vi "Preset GB VOLTAGE.vi"(8 "error in (no error)":errorcluster, 10 "Voltage":dbl=1.0 min=1.0 max=8.0 step=0.1 format="%.1f", 11 "VISA resource in":refnum<visa-resource-name>) -> (0 "error out":errorcluster, 3 "VISA resource out":refnum<visa-resource-name>)   [LabVIEW 2025, in "Chroma 19572.lvlib"]
doc: "This VI writes to the instrument the GFI state."
uses:
  <instrlib>/Chroma 19572/Chroma 19572.lvlib
panel:
  # "PreSet GB VOLTAGE"
  # "[V]"
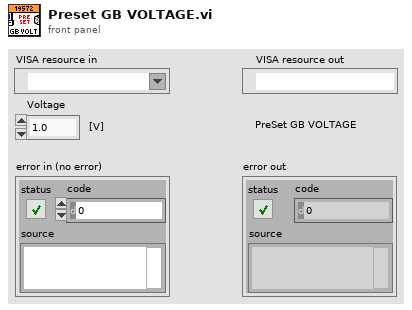
[diagram p1: front panel]
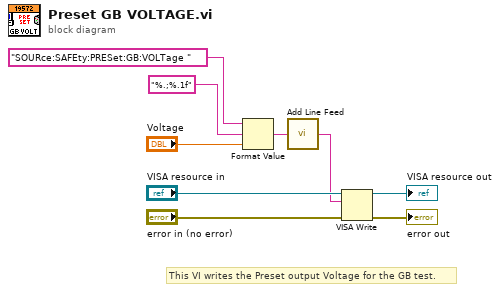
[diagram p0: block diagram]
diagram:
  # "This VI writes the Preset output Voltage for the GB test."
  n1 = Format Value(string ("")="SOURce:SAFEty:PRESet:GB:VOLTage ", format string="%.;%.1f", value (0)="Voltage") -> (output string=w3:string)
  n2 = call <instrlib>:"Add Line Feed.vi"("Command string"=w3) -> ("Concatenated string"=w2:string)  [unwired: 4 in]
  n3 = VISA Write(VISA resource name="VISA resource in", write buffer=w2, error in (no error)="error in (no error)") -> (VISA resource name out=→"VISA resource out":refnum<visa-resource-name>, error out=→"error out":errorcluster)  [unwired: 1 out]
